vi "Initialize.vi"(8 "error in (no error)":errorcluster, 9 "Reset (True)":bool=TRUE, 10 "ID Query (True)":bool=TRUE, 11 "VISA resource name":refnum<visa-resource-name>) -> (0 "error out":errorcluster, 3 "VISA resource name out":refnum<visa-resource-name>)   [LabVIEW 2020, in "PICOTEST M351XA Series.lvlib"]
doc: "Establishes communication with the instrument and optionally performs an instrument identification query and/or an instrument reset. It also places the instrument in a default state needed for other instrument driver operations. Therefore, call this VI before calling other instrument driver VIs for this instrument. Generally, you need to call the Initialize VI only once at the beginning of an application."
uses:
  PICOTEST M351XA Series.lvlib
panel:
  # "(c) 2009 PICOTEST CORP.  ALL RIGHTS RESERVED."
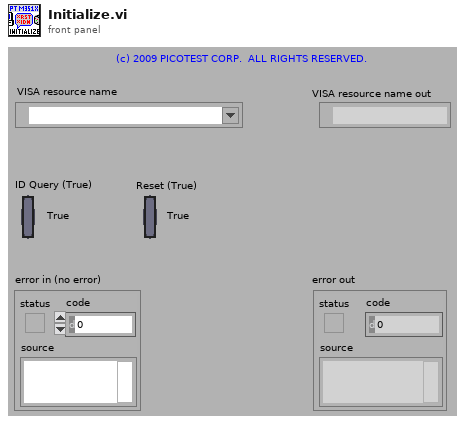
[diagram p1: front panel]
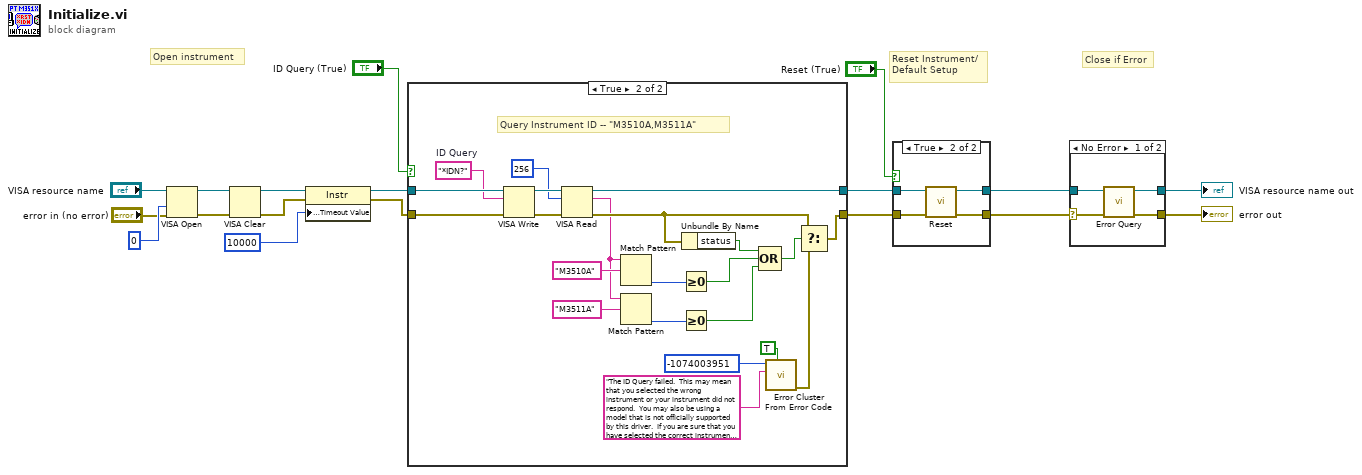
[diagram p0: block diagram]
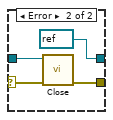
[diagram p2: hidden frame]
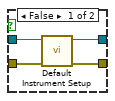
[diagram p3: hidden frame]
diagram:
  # "Close if Error"
  # "Reset Instrument/\nDefault Setup"
  # "Open instrument"
  n1 = VISA Open(access mode=u32 0, error in (no error)="error in (no error)", VISA resource name="VISA resource name") -> (VISA resource name=w11:refnum<visa-resource-name>, error out=w10:errorcluster)  [unwired: 2 in]
  n2 = VISA Clear(VISA resource name=w11, error in (no error)=w10) -> (VISA resource name out=w9:refnum<visa-resource-name>, error out=w8:errorcluster)
  n3 = property class="Instr"(reference=w9, error in=w8, "General Settings:Timeout Value"=u32 10000) -> (reference out=w3:refnum<visa-resource-name>, error out=w2:errorcluster)
  n4 = case shown="True" "ID Query (True)" {
    tunnel: [w19 w42] -> w17
    tunnel: [w20 w39] -> w18
    tunnel: w3 -> [w20 w40]
    tunnel: w2 -> [w19 w41]
    frame False {
    }
    frame True {
      w35 = "*IDN?"  # ID Query
      # "Query Instrument ID -- \"M3510A,M3511A\""
      n5 = VISA Write(VISA resource name=w40, write buffer=w35, error in (no error)=w41) -> (VISA resource name out=w38:refnum<visa-resource-name>, error out=w37:errorcluster)  [unwired: 1 out]
      n6 = VISA Read(VISA resource name=w38, byte count=u32 256, error in (no error)=w37) -> (VISA resource name out=w39:refnum<visa-resource-name>, read buffer=w21:string, error out=w30:errorcluster)  [unwired: 1 out]
      n7 = Match Pattern(string=w21, regular expression="M3510A") -> (offset past match=w28:i32)  [unwired: 1 in, 3 out]
      n8 = Match Pattern(string=w21, regular expression="M3511A") -> (offset past match=w25:i32)  [unwired: 1 in, 3 out]
      n9 = Greater Or Equal To 0?(x=w28) -> (x >= 0?=w27:bool)
      n10 = Greater Or Equal To 0?(x=w25) -> (x >= 0?=w24:bool)
      n11 = Unbundle By Name(w30) -> ("status"=w23:bool)
      n12 = Compound Arithmetic op=OR(w23, w27, w24) -> (w22:bool)
      n13 = call <vilib>:"Error Cluster From Error Code.vi"("show call chain? (False)"=TRUE, "error message (\"\")"="The ID Query failed.  This may mean that you selected the wrong instrument or your instrument did not respond.  You may also be using a model that is not officially supported by this driver.  If you are sure that you have selected the correct instrument and it is responding, try disabling the ID Query." ("Source (VI Name)"), "error code (0)"=-1074003951 ("Code")) -> ("error out"=w34:errorcluster)  [unwired: 6 in]
      n14 = Select(t=w30, s=w22, f=w34) -> (s? t:f=w42:errorcluster)
    }
  }
  n15 = case shown="True" "Reset (True)" {
    tunnel: w17 -> [w45 w47]
    tunnel: [w44 w50] -> w4
    tunnel: w18 -> [w46 w48]
    tunnel: [w43 w49] -> w5
    frame False {
      n16 = call "Default Instrument Setup.vi"("error in (no error)"=w45, "VISA resource name"=w46) -> ("error out"=w44:errorcluster, "VISA resource name out"=w43:refnum<visa-resource-name>)  [unwired: 8 in]
    }
    frame True {
      n17 = call "Reset.vi"("error in (no error)"=w47, "VISA resource name"=w48) -> ("error out"=w50:errorcluster, "VISA resource name out"=w49:refnum<visa-resource-name>)  [unwired: 8 in]
    }
  }
  n18 = case shown="No Error" w4 {
    selector: w4 -> [w52 w56]
    tunnel: w5 -> [w51 w57]
    tunnel: [w54 refnum<visa-resource-name> refnum ("VISA resource name out")] -> w7
    tunnel: [w53 w58] -> w6
    frame No Error {
      n19 = call "Error Query.vi"("error in (no error)"=w52, "VISA resource name"=w51) -> ("error out"=w53:errorcluster, "VISA resource name out"=w54:refnum<visa-resource-name>)  [unwired: 6 in, 2 out]
    }
    frame Error {
      n20 = call "Close.vi"("error in (no error)"=w56, "VISA resource name"=w57) -> ("error out"=w58:errorcluster)  [unwired: 9 in]
    }
  }
  "VISA resource name out" <- w7
  "error out" <- w6
